vi "例5-1.vi"() -> ()   [LabVIEW 2019]
uses:
  <vilib>/DAQmx/read.llb/DAQmx Read (Analog Wfm 1Chan NSamp).vi
  <vilib>/DAQmx/create/channels.llb/DAQmx Create Channel (AI-Voltage-Basic).vi
  <vilib>/DAQmx/configure/timing.llb/DAQmx Timing (Sample Clock).vi
  <vilib>/DAQmx/miscellaneous.llb/DAQmx Fill In Error Info.vi
panel:
  out "波形图":waveform(dbl)(graph)
  in  "samples per channel":i32=100 caption="每通道采样"
  in  "rate":dbl=1000.0 caption="速率" format="%0.2f"
  in  "minimum value":dbl=-5.0 caption="最小值" format="%0.2f"
  in  "maximum value":dbl=5.0 caption="最大值" format="%0.2f"
  in  "physical channels":tag caption="物理通道"
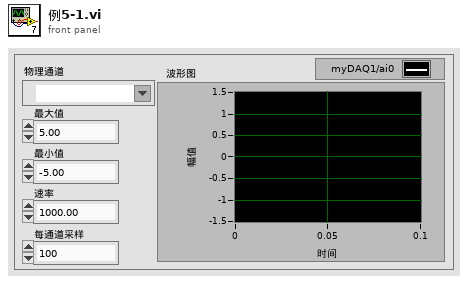
[diagram p1: front panel]
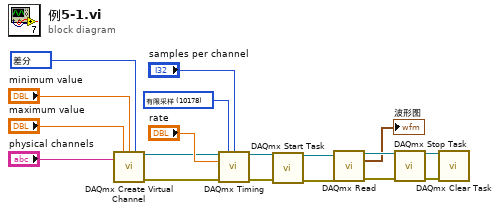
[diagram p0: block diagram]
diagram:
  w13 = 10178 items=["有限采样"=10178, "连续采样"=10123, "硬件定时单点"=12522] ("sample mode")
  w15 = 10106 items=["默认"=-1, "RSE"=10083, "NRSE"=10078, "差分"=10106, "伪差分"=12529] ("input terminal configuration")
  n1 = call-poly <vilib>:"DAQmx Create Virtual Channel.vi"("maximum value"="maximum value", "minimum value"="minimum value", "input terminal configuration"=w15, "physical channels"="physical channels") -> ("task out"=w11:refnum<k21>, "error out"=w9:errorcluster)  [unwired: 10 in]
  n2 = call-poly <vilib>:"DAQmx Timing.vi"("task/channels in"=w11, "sample mode"=w13, "samples per channel"="samples per channel", "rate"="rate", "error in"=w9) -> ("task out"=w10:refnum<k21>, "error out"=w8:errorcluster)  [unwired: 9 in]
  n3 = call <vilib>:"DAQmx Start Task.vi"("task/channels in"=w10, "error in"=w8) -> ("task out"=w7:refnum<k21>, "error out"=w6:errorcluster)  [unwired: 12 in]
  n4 = call-poly <vilib>:"DAQmx Read.vi"("task/channels in"=w7, "error in"=w6) -> ("task out"=w5:refnum<k21>, "data"=→"波形图":waveform(dbl), "error out"=w4:errorcluster)  [unwired: 11 in]
  n5 = call <vilib>:"DAQmx Stop Task.vi"("task/channels in"=w5, "error in"=w4) -> ("task out"=w3:refnum<k21>, "error out"=w2:errorcluster)  [unwired: 12 in]
  n6 = call <vilib>:"DAQmx Clear Task.vi"("task in"=w3, "error in"=w2) -> ()  [unwired: 13 in, 1 out]
